vi "niScope LabVIEW Error.vi"(2 "instrument handle":u32, 3 "niScope error code (0)":i32 format="%.0x", 5 "error in (no error)":errorcluster) -> (1 "error out":errorcluster)   [LabVIEW 2020]
uses:
  niScope_32.dll
panel:
  out "VI Name":string
  out "instrument handle out":i32
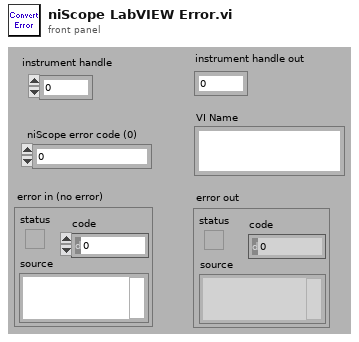
[diagram p1: front panel]
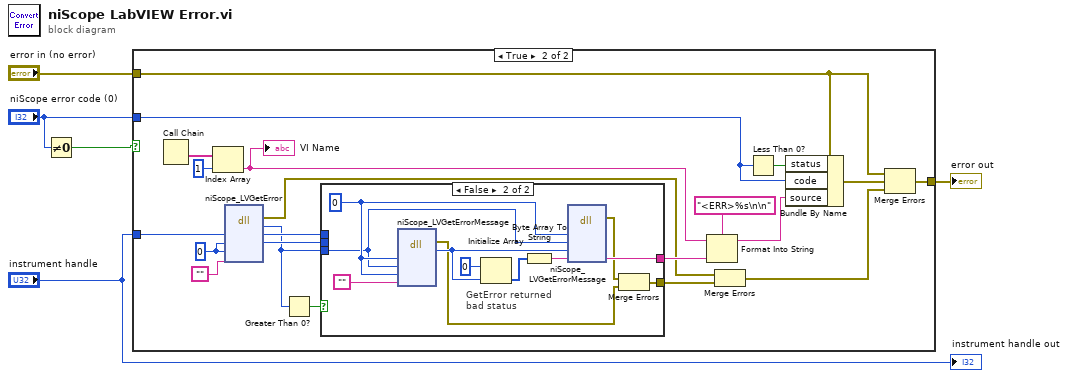
[diagram p0: block diagram]
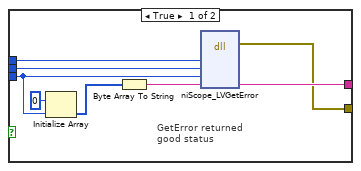
[diagram p3: hidden frame]
diagram:
  n1 = Not Equal To 0?(x="niScope error code (0)") -> (x != 0?=w1:bool)
  n2 = case shown="True" w1 {
    tunnel: "niScope error code (0)" -> [_ w18]
    tunnel: [w6 w14] -> w5
    tunnel: "instrument handle" -> [_ w17]
    tunnel: "error in (no error)" -> [w6 w16]
    frame False {
    }
    frame True {
      w24 = 0
      n3 = Call Chain() -> (call chain=w25:string[])
      n4 = Index Array(array=w25, index=1 ("Index")) -> (element=w10:string)
      "VI Name" <- w10
      n5 = dll-call lib="niScope_*.*" fn="niScope_LVGetError" label="GetError"("instrumentHandle"=w17, "errorCode"=w24, "bufferSize"=w24, "description"="") -> (error out=w8:errorcluster, w11:i32, "instrumentHandle"=w23:u32, "errorCode"=w22:i32)  [unwired: 5 in, 1 out]
      n6 = Greater Than 0?(x=w11) -> (x > 0?=w12:bool)
      n7 = case shown="False" w12 {
        tunnel: w23 -> [w32 _]
        tunnel: w22 -> [w31 _]
        tunnel: [w30 w46] -> w21
        tunnel: w11 -> [w29 w43]
        tunnel: [w28 w38] -> w9
        frame True {
          # "GetError returned\ngood status"
          n8 = Initialize Array(u8 0, w29) -> (w34:u8[])
          n9 = Byte Array To String(unsigned byte array=w34) -> (string=w33:string)
          n10 = dll-call lib="niScope_*.*" fn="niScope_LVGetError" label="GetError"("instrumentHandle"=w32, "errorCode"=w31, "bufferSize"=w29, "description"=w33) -> (error out=w28:errorcluster, "description"=w30:string)  [unwired: 7 in, 1 out]
        }
        frame False {
          w45 = 0 ("instrumentHandle")
          # "GetError returned\nbad status"
          n11 = dll-call lib="niScope_*.*" fn="niScope_LVGetErrorMessage" label="GetErrorMessage"("instrumentHandle"=w45, "errorCode"=w43, "bufferSize"=w45, "errorMessage"="") -> (error out=w36:errorcluster, w39:i32)  [unwired: 7 in, 1 out]
          n12 = Initialize Array(u8 0, w39) -> (w42:u8[])
          n13 = Byte Array To String(unsigned byte array=w42) -> (string=w40:string)
          n14 = dll-call lib="niScope_*.*" fn="niScope_LVGetErrorMessage" label="GetErrorMessage"("instrumentHandle"=w45, "errorCode"=w43, "bufferSize"=w39, "errorMessage"=w40) -> (error out=w37:errorcluster, "errorMessage"=w46:string)  [unwired: 7 in, 1 out]
          n15 = Merge Errors(w37, w36) -> (w38:errorcluster)
        }
      }
      n16 = Format Into String(format string="<ERR>%s\n\n", initial string=w10, w21) -> (resulting string=w13:string)  [unwired: 1 in, 1 out]
      n17 = Merge Errors(w8, w9) -> (w7:errorcluster)
      n18 = Less Than 0?(x=w18) -> (x < 0?=w27:bool)
      n19 = Bundle By Name(cluster=w16, "status"=w27, "code"=w18, "source"=w13) -> (w15:errorcluster)
      n20 = Merge Errors(w16, w15, w7) -> (w14:errorcluster)
    }
  }
  "error out" <- w5
  "instrument handle out" <- "instrument handle"
